vi "Write Display Type.vi"(10 "Display Type":T1, 11 "Assert Display in":refnum<class "Assert Display.lvclass">) -> (3 "Assert Display out":refnum<class "Assert Display.lvclass">)   [LabVIEW 2016, in "Assert API Components.lvlib" / "Assert Display.lvlib" / "Assert Display.lvclass"]
uses:
  Assert Display.lvclass
  Assert API Components/Display Type.ctl
  Assert Display.lvclass/Assert Display.ctl
  Assert API Components/Assert API Components.lvlib
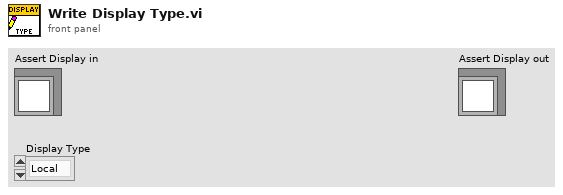
[diagram p1: front panel]
types:
  T1 = typedef "Assert API Components.lvlib/Display Type.ctl" = enum16{"Local", "Network"}
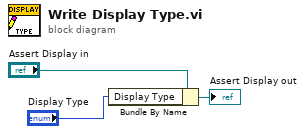
[diagram p0: block diagram]
diagram:
  n1 = Bundle By Name(cluster="Assert Display in", "Display Type"="Display Type") -> (→"Assert Display out":refnum<class "Assert Display.lvclass">)
